vi "MTS_RGBToU32.vi"(9 "Blue":u8, 10 "Green":u8, 11 "Red":u8) -> (2 "Color":u32)   [LabVIEW 2011]
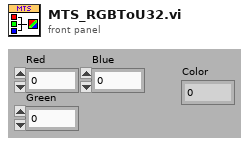
[diagram p1: front panel]
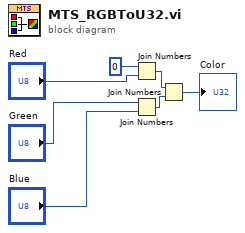
[diagram p0: block diagram]
diagram:
  n1 = Join Numbers(hi=u8 0, lo="Red") -> ((hi.lo)=w6:u16)
  n2 = Join Numbers(hi="Green", lo="Blue") -> ((hi.lo)=w7:u16)
  n3 = Join Numbers(hi=w6, lo=w7) -> ((hi.lo)=→"Color":u32)
